vi "SpreadsheetFGV.vi"(7 "FGV Control":T1, 8 "Error In":errorcluster, 10 "Check -in Time":timestamp, 11 "Student ID":i32) -> (0 "Error Out":errorcluster, 1 "Checked In?":bool, 2 "Names":string[](array[string]), 3 "Message":string, 4 "Elapsed Time":i32)   [LabVIEW 2013]
uses:
  Controls/CSVFGVStates.ctl
  <vilib>/Utility/file.llb/Write To Spreadsheet File (string).vi
  <vilib>/Utility/file.llb/Read From Spreadsheet File (string).vi
panel:
  out "Output 2D Data":string[][](array[string])
  in  "CheckedInOutColumn":i32=3
  out "Checked In":string
  out "all rows":string[][](array[string])
  in  "Replacement":string
  in  "Student Names":i32(listbox)
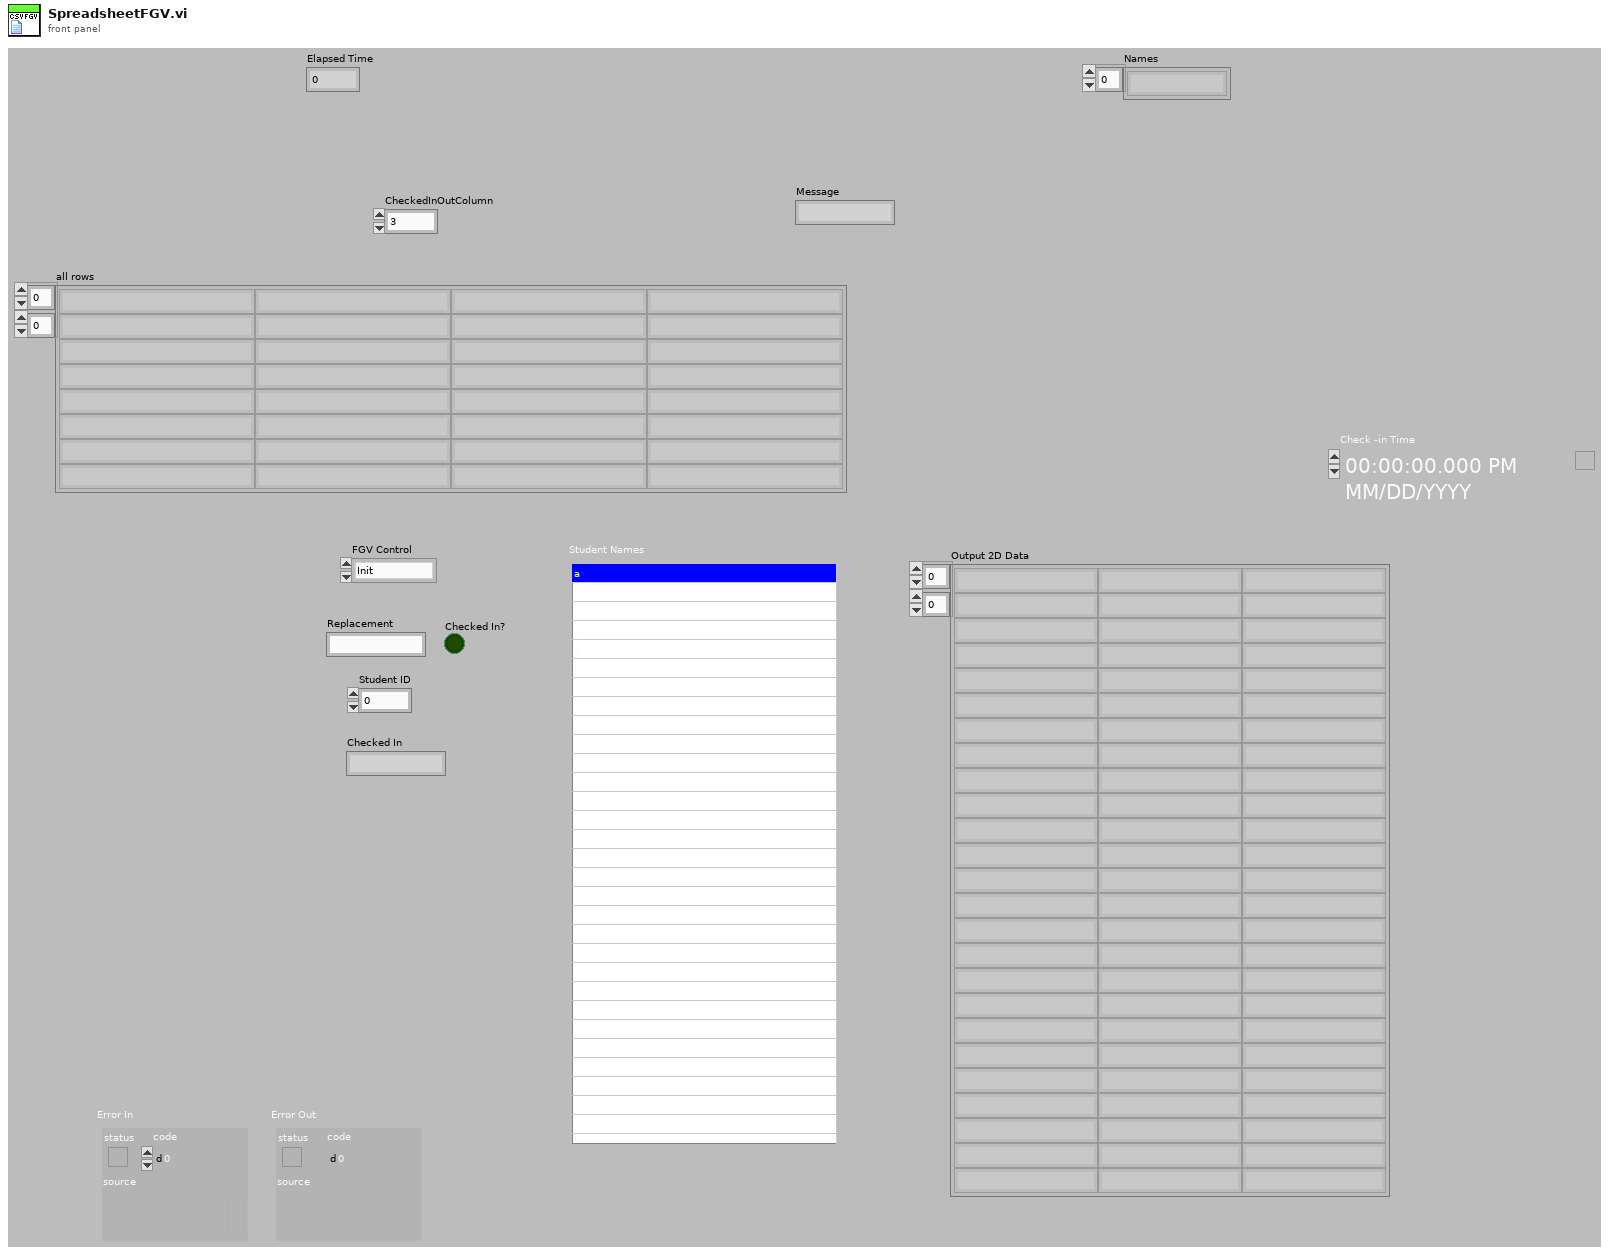
[diagram p1: front panel]
types:
  T1 = typedef "CSVFGVStates.ctl" = enum16{"Init", "Sort", "Check In", "Check Out", "Check Status", "Read CSV", "Close Out"}
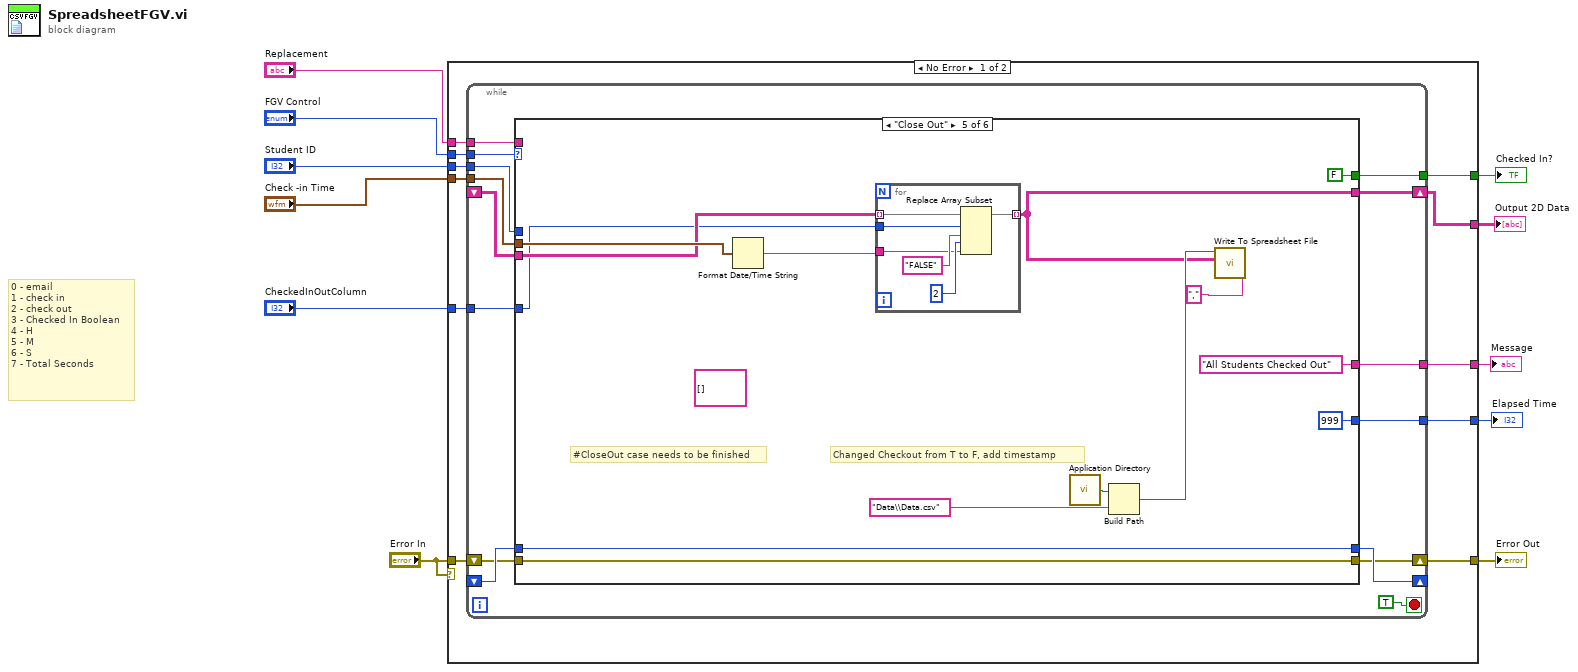
[diagram p0: block diagram]
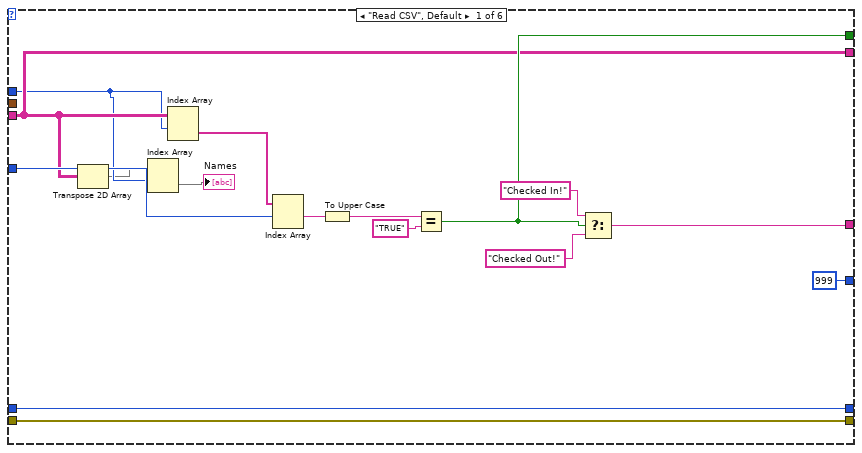
[diagram p2: hidden frame]
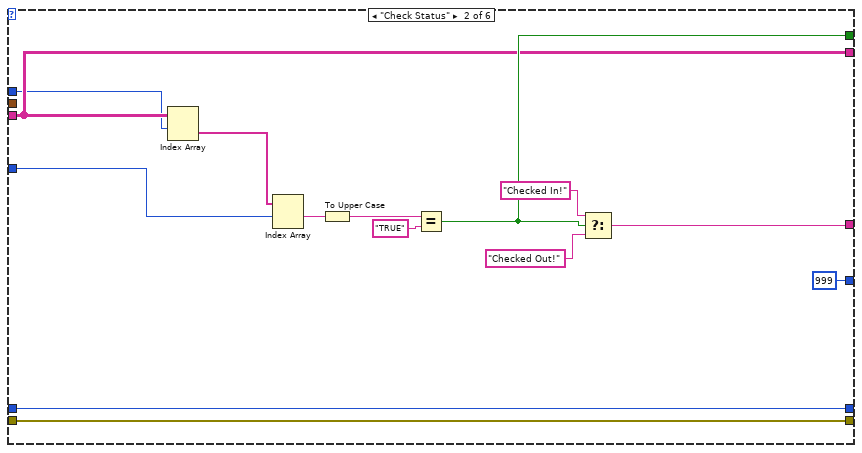
[diagram p3: hidden frame]
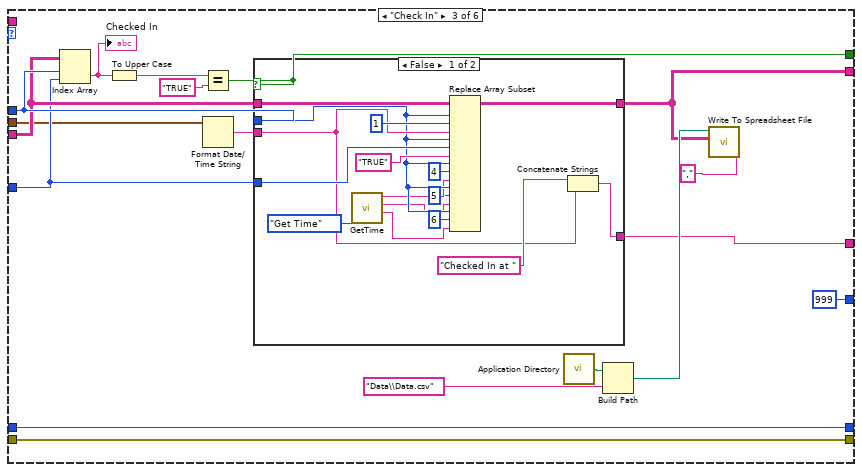
[diagram p4: hidden frame]
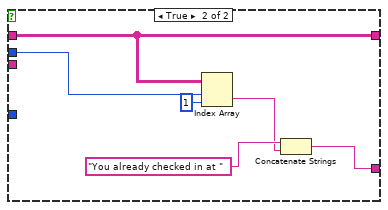
[diagram p5: hidden frame]
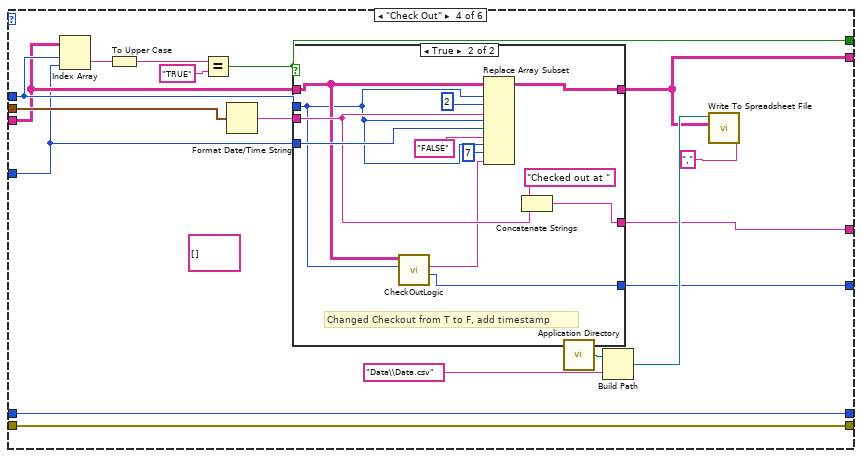
[diagram p6: hidden frame]
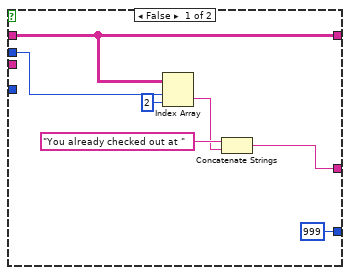
[diagram p7: hidden frame]
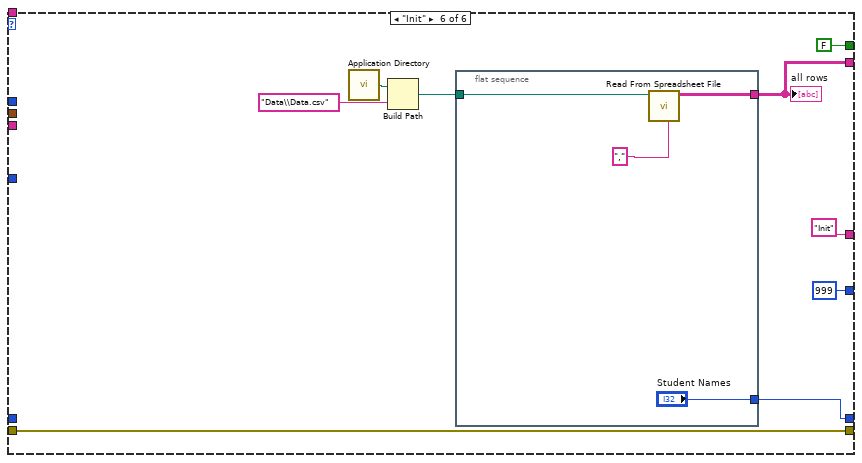
[diagram p8: hidden frame]
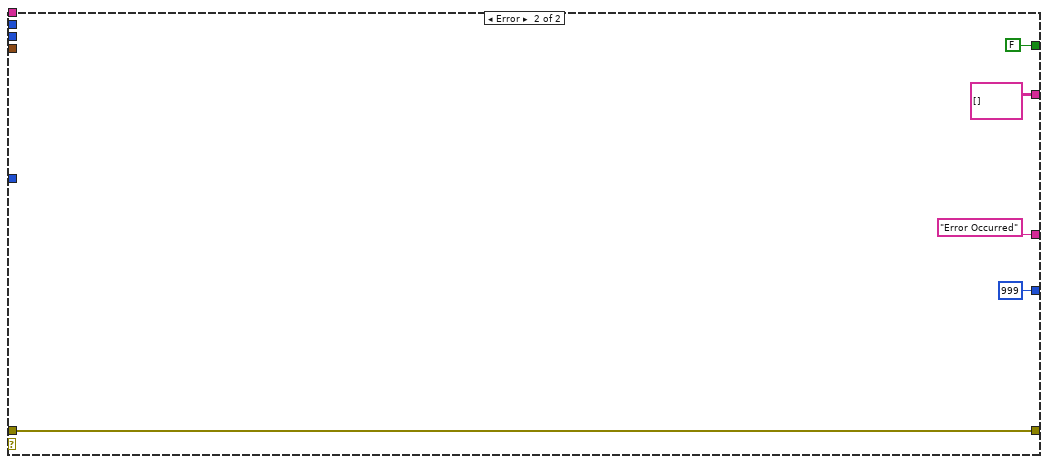
[diagram p9: hidden frame]
diagram:
  # "0 - email\n1 - check in\n2 - check out\n3 - Checked In Boolean\n4 - H\n5 - M\n6 - S\n7 - Total Seconds"
  n1 = case shown="No Error" "Error In" {
    tunnel: "FGV Control" -> [w22 _]
    tunnel: "Error In" -> [w20 w182]
    tunnel: [w21 w182] -> w9
    tunnel: "Student ID" -> [w19 _]
    tunnel: "Check -in Time" -> [w18 _]
    tunnel: "Replacement" -> [w17 _]
    tunnel: [w16 FALSE] -> w5
    tunnel: "CheckedInOutColumn" -> [w15 _]
    tunnel: [w14 string[][] [] ("all rows")] -> w3
    tunnel: [w13 "Error Occurred" ("date/time string")] -> w2
    tunnel: [w12 999 ("Elapsed Seconds")] -> w1
    frame No Error {
      n2 = while {
        shift-right: [w27] -> w14
        shift-left: _ -> [w35]
        tunnel: w22 -> [w36]
        shift-right: [w34] -> _
        shift-left: _ -> [w33]
        shift-right: [w32] -> w21
        shift-left: w20 -> [w31]
        tunnel: w19 -> [w30]
        tunnel: w18 -> [w29]
        tunnel: w17 -> [w28]
        tunnel: [w26] -> w16
        tunnel: w15 -> [w25]
        tunnel: [w24] -> w13
        tunnel: [w23] -> w12
        stop <- TRUE stop-if-true
        n3 = case shown="\"Close Out\"" w36 {
          tunnel: w35 -> [w41 w55 w73 w112 w150 _]
          tunnel: [w52 w66 w81 w121 w154 w171] -> w34
          tunnel: w33 -> [w52 w66 w81 w121 w154 _]
          tunnel: [w53 w67 w83 w123 w156 w170] -> w32
          tunnel: w31 -> [w53 w67 w83 w123 w156 w170]
          tunnel: w30 -> [w40 w54 w74 w113 _ _]
          tunnel: w29 -> [_ _ w69 w119 w152 _]
          tunnel: w28 -> [_ _ _ _ _ _]
          tunnel: [w41 w55 w78 w117 w151 w169] -> w27
          tunnel: [w45 w59 w72 w111 FALSE FALSE] -> w26
          tunnel: w25 -> [w46 w60 w70 w110 w149 _]
          tunnel: [w42 w56 w71 w109 "All Students Checked Out" ("date/time string") "Init" ("date/time string")] -> w24
          tunnel: [999 ("Elapsed Seconds") 999 ("Elapsed Seconds") 999 ("Elapsed Seconds") w108 999 ("Elapsed Seconds") 999 ("Elapsed Seconds")] -> w23
          frame "Read CSV", Default {
            n4 = Transpose 2D Array(2D array=w41) -> (transposed array=w39:string[][])
            n5 = Index Array(array=w39, index (row)=w40) -> (element=→"Names":string[])  [unwired: 1 in]
            n6 = Index Array(array=w41, index (row)=w40) -> (element=w47:string[])  [unwired: 1 in]
            n7 = Index Array(array=w47, index #1=w46) -> (element #1=w50:string)  [unwired: 1 in, 1 out]
            n8 = To Upper Case(1:w50) -> (0:w49:string)
            n9 = Equal?(x=w49, y="TRUE") -> (x = y?=w45:bool)
            n10 = Select(t="Checked In!" ("y"), s=w45, f="Checked Out!" ("y")) -> (s? t:f=w42:string)
          }
          frame "Check Status" {
            n11 = Index Array(array=w55, index (row)=w54) -> (element=w61:string[])  [unwired: 1 in]
            n12 = Index Array(array=w61, index #1=w60) -> (element #1=w64:string)  [unwired: 1 in, 1 out]
            n13 = To Upper Case(1:w64) -> (0:w63:string)
            n14 = Equal?(x=w63, y="TRUE") -> (x = y?=w59:bool)
            n15 = Select(t="Checked In!" ("y"), s=w59, f="Checked Out!" ("y")) -> (s? t:f=w56:string)
          }
          frame "Check In" {
            n16 = Index Array(array=w73, index (row)=w74, index (col)=w70) -> (element=w77:string)
            "Checked In" <- w77
            n17 = To Upper Case(1:w77) -> (0:w76:string)
            n18 = Equal?(x=w76, y="TRUE") -> (x = y?=w72:bool)
            n19 = Format Date/Time String(seconds (now)=w69) -> (date/time string=w79:string)  [unwired: 2 in]
            n20 = case shown="False" w72 {
              tunnel: w79 -> [w95 _]
              tunnel: [w100 w107] -> w78
              tunnel: w74 -> [w93 w106]
              tunnel: w73 -> [w98 w107]
              tunnel: [w94 w102] -> w71
              tunnel: w70 -> [w97 _]
              frame False {
                n21 = call "GetTime.vi"("State"=enum16{"Get Time", "Calculate Differential"}."Get Time") -> ("Seconds"=w87:string, "Minutes"=w89:string, "Hours"=w91:string)  [unwired: 5 in, 3 out]
                n22 = Replace Array Subset(array=w98, new element #1=w95, index (row) #1=w93, index (col) #1=1 ("disabled index (col)"), new element #2="TRUE" ("new element/subarray"), index (row) #2=w93, index (col) #2=w97, new element #3=w91, index (row) #3=w93, index (col) #3=4 ("disabled index (col)"), new element #4=w89, index (row) #4=w93, index (col) #4=5 ("disabled index (col)"), new element #5=w87, index (row) #5=w93, index (col) #5=6 ("disabled index (col)")) -> (w100:string[][])
                n23 = Concatenate Strings("Checked In at " ("String"), w95) -> (w94:string)
              }
              frame True {
                n24 = Index Array(array=w107, index (row)=w106, index (col)=1 ("disabled index (col)")) -> (element=w103:string)
                n25 = Concatenate Strings("You already checked in at " ("delimiter (\\t)"), w103) -> (w102:string)
              }
            }
            n26 = call <vilib>:"Application Directory.vi"() -> ("Application Directory"=w85:path)
            n27 = Build Path(base path=w85, name or relative path="Data\\Data.csv") -> (appended path=w82:path)
            n28 = call-poly <vilib>:"Write To Spreadsheet File.vi"("delimiter (\\t)"="," ("delimiter (\\t)"), "2D data"=w78, "file path (dialog if empty)"=w82) -> ()  [unwired: 5 in, 1 out]
          }
          frame "Check Out" {
            (unwired) string[][] [] ("all rows")
            n29 = Index Array(array=w112, index (row)=w113, index (col)=w110) -> (element=w116:string)
            n30 = To Upper Case(1:w116) -> (0:w115:string)
            n31 = Equal?(x=w115, y="TRUE") -> (x = y?=w111:bool)
            n32 = Format Date/Time String(seconds (now)=w119) -> (date/time string=w118:string)  [unwired: 2 in]
            n33 = case shown="True" w111 {
              tunnel: w118 -> [_ w140]
              tunnel: [w132 w143] -> w117
              tunnel: w113 -> [w131 w136]
              tunnel: w112 -> [w132 w137]
              tunnel: [w127 w139] -> w109
              tunnel: w110 -> [_ w141]
              tunnel: [999 ("Elapsed Seconds") w133] -> w108
              frame False {
                n34 = Index Array(array=w132, index (row)=w131, index (col)=2 ("disabled index (col)")) -> (element=w128:string)
                n35 = Concatenate Strings("You already checked out at " ("string"), w128) -> (w127:string)
              }
              frame True {
                # "Changed Checkout from T to F, add timestamp"
                n36 = call "CheckOutLogic.vi"("Student ID"=w136, "all rows"=w137) -> ("Total Elapsed Time"=w133:i32, "Total Seconds Out"=w134:string)  [unwired: 7 in, 1 out]
                n37 = Replace Array Subset(array=w137, new element #1=w140, index (row) #1=w136, index (col) #1=2 ("disabled index (col)"), new element #2="FALSE" ("new element/subarray"), index (row) #2=w136, index (col) #2=w141, new element #3=w134, index (row) #3=w136, index (col) #3=7 ("disabled index (col)")) -> (w143:string[][])
                n38 = Concatenate Strings("Checked out at " ("string"), w140) -> (w139:string)
              }
            }
            n39 = call <vilib>:"Application Directory.vi"() -> ("Application Directory"=w125:path)
            n40 = Build Path(base path=w125, name or relative path="Data\\Data.csv") -> (appended path=w122:path)
            n41 = call-poly <vilib>:"Write To Spreadsheet File.vi"("delimiter (\\t)"="," ("delimiter (\\t)"), "2D data"=w117, "file path (dialog if empty)"=w122) -> ()  [unwired: 5 in, 1 out]
          }
          frame "Close Out" {
            (unwired) string[][] [] ("all rows")
            # "#CloseOut case needs to be finished"
            # "Changed Checkout from T to F, add timestamp"
            n42 = Format Date/Time String(seconds (now)=w152) -> (date/time string=w146:string)  [unwired: 2 in]
            n43 = for {
              tunnel: [w164] -> w151 mode=indexing
              tunnel: w150 -> [w163] mode=indexing
              tunnel: w149 -> [w162]
              tunnel: w146 -> [w159]
              n44 = Replace Array Subset(array=w163, new element #1="FALSE" ("new element/subarray"), index #1=w162, new element #2=w159, index #2=2 ("index")) -> (w164:string[])
            }
            n45 = call <vilib>:"Application Directory.vi"() -> ("Application Directory"=w158:path)
            n46 = Build Path(base path=w158, name or relative path="Data\\Data.csv") -> (appended path=w155:path)
            n47 = call-poly <vilib>:"Write To Spreadsheet File.vi"("delimiter (\\t)"="," ("delimiter (\\t)"), "2D data"=w151, "file path (dialog if empty)"=w155) -> ()  [unwired: 5 in, 1 out]
          }
          frame "Init" {
            n48 = call <vilib>:"Application Directory.vi"() -> ("Application Directory"=w173:path)
            n49 = Build Path(base path=w173, name or relative path="Data\\Data.csv") -> (appended path=w168:path)
            n50 = flat-sequence {
              tunnel: w168 -> [w177]
              tunnel: [w176] -> w169
              tunnel: ["Student Names"] -> w171
              frame #0 {
                n51 = call-poly <vilib>:"Read From Spreadsheet File.vi"("delimiter (\\t)"="," ("delimiter (\\t)"), "file path (dialog if empty)"=w177) -> ("all rows"=w176:string[][])  [unwired: 5 in, 4 out]
              }
            }
            "all rows" <- w169
          }
        }
      }
    }
    frame Error {
    }
  }
  "Error Out" <- w9
  "Checked In?" <- w5
  "Output 2D Data" <- w3
  "Message" <- w2
  "Elapsed Time" <- w1
